vi "Buffer Setpoints.vi"(8 "error in (no error)":errorcluster, 11 "Model in":refnum<class "Model.lvclass">) -> (0 "error out":errorcluster, 3 "Model out":refnum<class "Model.lvclass">)   [LabVIEW 2016, in "Model.lvclass"]
uses:
  Model.lvclass
  Model.lvclass/Model.ctl
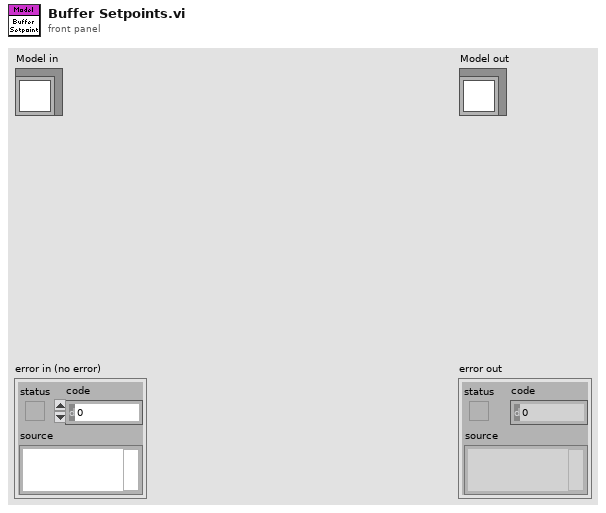
[diagram p1: front panel]
types:
  T1 = typedef "FAMT Typedefs.lvlib/ActuatorSetPoints.ctl" = cluster{"Axial Force":dbl, "Lateral Force":dbl, "FC1 Force":dbl, "FC2 Force":dbl}
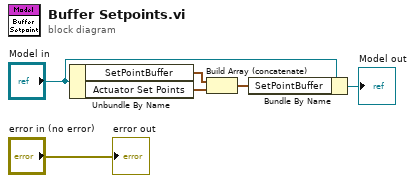
[diagram p0: block diagram]
diagram:
  n1 = Unbundle By Name("Model in") -> ("SetPointBuffer"=w6:T1[], "Actuator Set Points"=w5:T1)
  n2 = Build Array (concatenate)(w6, w5) -> (w3:T1[])
  n3 = Bundle By Name(cluster="Model in", "SetPointBuffer"=w3) -> (→"Model out":refnum<class "Model.lvclass">)
  "error out" <- "error in (no error)"
